vi "io-find-by-name.vi"(10 "IO Name":string, 11 "IO Nodes in":T1[](array[typedef]) {"calibration"."Y" format="%#.3f"; "calibration"."X" format="%#.3f"; "ADDR" format="%04d"}) -> (0 "Found?":bool, 1 "Last Index":i32, 3 "IO Nodes out":T1[](array[typedef]) {"calibration"."Y" format="%#.3f"; "calibration"."X" format="%#.3f"; "ADDR" format="%04d"})   [LabVIEW 2024]
uses:
  controls/IONode.ctl
  controls/type.address.ctl
  controls/enum.io.type.ctl
  controls/enum.io.mode.ctl
  controls/typeXyPoint.ctl
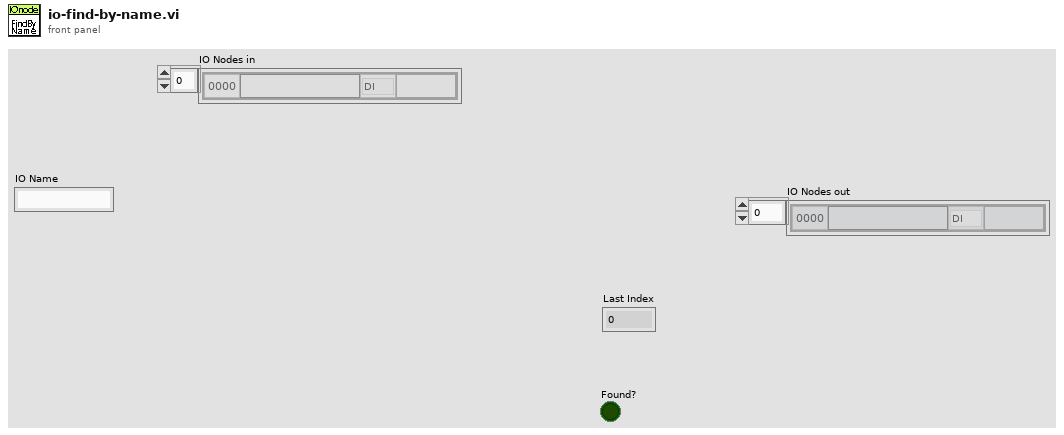
[diagram p1: front panel]
types:
  T1 = typedef "IONode.ctl" = cluster{"ADDR":T2, "Label":string, "Type":T3, "Mode":T4, "Value":string, "Tags":string, "calibration":T5[]}
  T2 = typedef "type.address.ctl" = u16
  T3 = typedef "enum.io.type.ctl" = enum16{"Type", "DI", "DO", "AI", "AO", "VL", "BUF"}
  T4 = typedef "enum.io.mode.ctl" = enum16{"Mode", "RIO", "SIM"}
  T5 = typedef "typeXyPoint.ctl" = cluster{"X":dbl, "Y":dbl}
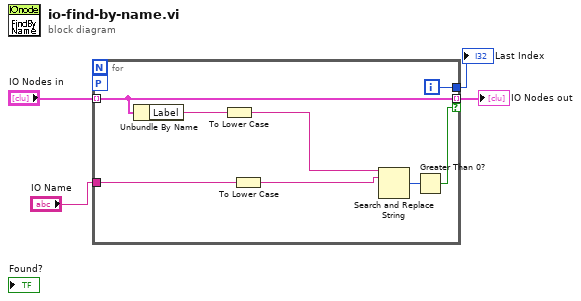
[diagram p0: block diagram]
diagram:
  n1 = for {
    tunnel: "IO Nodes in" -> [w11] mode=indexing
    tunnel: "IO Name" -> [w9]
    tunnel: [w12] -> w3
    tunnel: [w11] -> w1 mode=indexing if=w7
    workers-P: _ -> [_]
    i -> [w12]
    n2 = Unbundle By Name(w11) -> ("Label"=w10:string)
    n3 = To Lower Case(string=w10) -> (all lower case string=w6:string)
    n4 = To Lower Case(string=w9) -> (all lower case string=w5:string)
    n5 = Search and Replace String(input string=w6, search string=w5) -> (number of replacements=w8:i32)  [unwired: 6 in, 3 out]
    n6 = Greater Than 0?(x=w8) -> (x > 0?=w7:bool)
  }
  "IO Nodes out" <- w1
  "Last Index" <- w3
